vi "Handle Last Ack Core.vi"(4 "error in (no error)":errorcluster, 6 "Last Ack":refnum<class "Last Ack.lvclass">, 7 "Worker in":refnum<class "Worker Actor.lvclass">) -> (0 "error out":errorcluster, 3 "Worker out":refnum<class "Worker Actor.lvclass">)   [LabVIEW 2021, in "Worker Actor.lvclass"]
doc: "(<B>Filename</B>: Actor Framework.lvlib:Actor.lvclass:Handle Last Ack Core.vi)\n\nDefines how the caller actor responds to the Last Ack message from a nested actor. The Last Ack message is the final message a nested actor sends to its caller before it shuts down. The message contains information about the final state of the nested actor.\n\nBy default, this method does nothing except return any error the nested actor sent. A descendant class may override this method to define behavior."
uses:
  Worker Actor.lvclass
  Template Module/Template Module.lvclass
  Loggers/Logger/Logger.lvclass
  <vilib>/ActorFramework/LastAck/Last Ack.lvclass
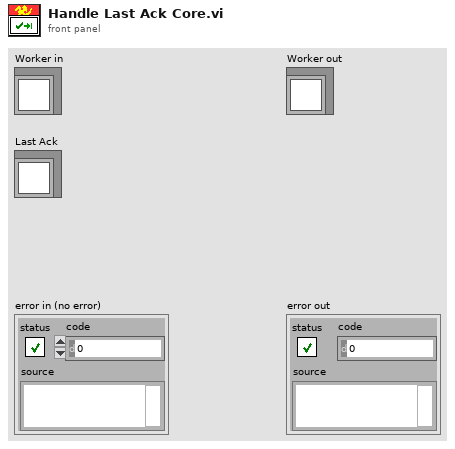
[diagram p1: front panel]
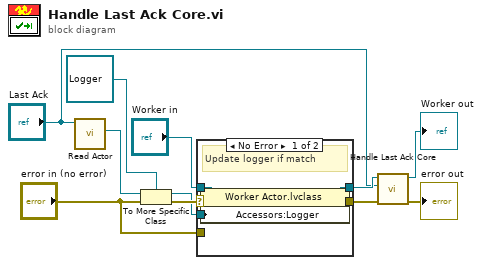
[diagram p0: block diagram]
diagram:
  n1 = call <vilib>:"Read Actor.vi"("Last Ack"="Last Ack") -> ("Actor"=w1:refnum<class "Actor.lvclass">)  [unwired: 10 in]
  n2 = To More Specific Class(target class=refnum<class "Logger.lvclass"> refnum ("Logger.lvclass"), reference=w1, error in="error in (no error)") -> (specific class reference=w6:refnum<class "Logger.lvclass">, error out=w8:errorcluster)
  n3 = case shown="No Error" w8 {
    selector: w8 -> [w15 _]
    tunnel: "Worker in" -> [w16 w18]
    tunnel: w6 -> [w14 _]
    tunnel: [w13 w18] -> w4
    tunnel: [w12 w17] -> w3
    tunnel: "error in (no error)" -> [_ w17]
    frame No Error {
      # "Update logger if match"
      n4 = property class="Worker Actor.lvclass"(reference=w16, error in=w15, "Accessors:Logger"=w14) -> (reference out=w13:refnum<class "Worker Actor.lvclass">, error out=w12:errorcluster)
    }
    frame Error {
    }
  }
  n5 = call-parent "Handle Last Ack Core.vi"("error in (no error)"=w3, "Last Ack"="Last Ack", "Actor in"=w4) -> ("error out"=→"error out":errorcluster, "Actor out"=→"Worker out":refnum<class "Worker Actor.lvclass">)  [unwired: 3 in]
